vi "Analyze Frequency Response.vi"(0 "Per-Frequency Per-Site Waveform In":waveform(dbl)[][](array[waveform]), 5 "Frequency (Hz)":dbl[](array[numeric]), 7 "Window(Rectangle)":T1(ring), 11 "error in (no error)":errorcluster) -> (4 "DC values(V)":dbl[][](array[numeric]), 6 "detected amplitudes(Unit Peak)":dbl[][](array[numeric]), 8 "detected phases (deg)":dbl[][](array[numeric]), 10 "THD(%)":dbl[][](array[numeric]), 15 "error out":errorcluster)   [LabVIEW 2020]
doc: "This Vi helps to calculate the frequency response such as Amplitude, THD, Phase and DC Offset for the DUT or Ref_Mic"
uses:
  <vilib>/measure/matone.llb/Harmonic Distortion Analyzer N Chan.vi
  <vilib>/measure/matone.llb/Extract Single Tone Information N Chan.vi
  <vilib>/measure/madcrms.llb/Basic Averaged DC-RMS for N Chan.vi
  <vilib>/measure/NI_MAPro.lvlib
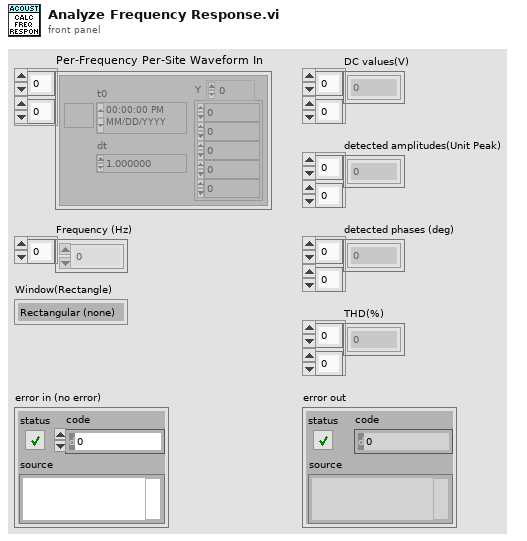
[diagram p1: front panel]
types:
  T1 = enum16{"Rectangular (none)", "Hanning", "Low side lobe"}
  T2 = cluster{"approx freq. (optional)":dbl, "search (+/- % of Fsampl.)":dbl}
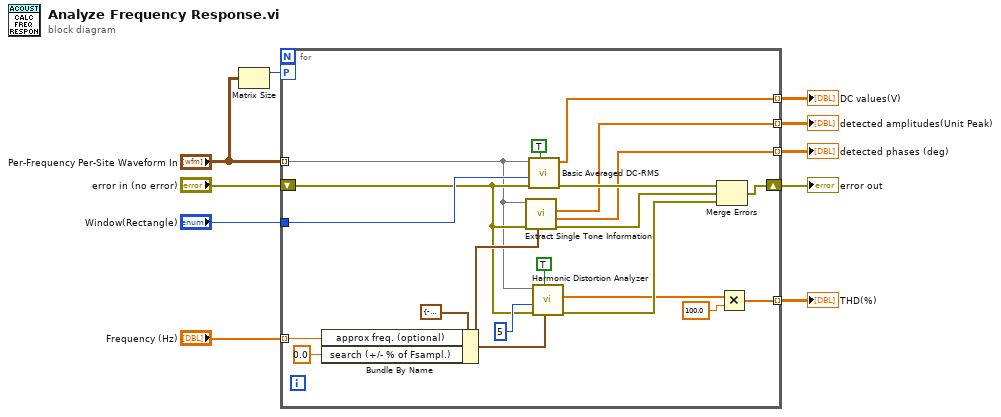
[diagram p0: block diagram]
diagram:
  n1 = Matrix Size(0:"Per-Frequency Per-Site Waveform In") -> (1:w1:i32)  [unwired: 1 out]
  n2 = for {
    tunnel: "Window(Rectangle)" -> [w25]
    shift-right: [w17] -> w8
    shift-left: "error in (no error)" -> [w23]
    tunnel: "Frequency (Hz)" -> [w21] mode=indexing
    tunnel: "Per-Frequency Per-Site Waveform In" -> [w22] mode=indexing
    tunnel: [w16] -> w6 mode=indexing
    tunnel: [w15] -> w5 mode=indexing
    tunnel: [w14] -> w4 mode=indexing
    tunnel: [w11] -> w3 mode=indexing
    workers-P: w1 -> [_]
    n3 = Bundle By Name(cluster=T2 {"approx freq. (optional)"=-1.0, "search (+/- % of Fsampl.)"=5.0} ("advanced search"), "approx freq. (optional)"=w21, "search (+/- % of Fsampl.)"=0.0) -> (w26:T2)
    n4 = call-poly <vilib>:"Extract Single Tone Information.vi"("advanced search"=w26, "error in (no error)"=w23, "time signals in"=w22) -> ("error out"=w19:errorcluster, "detected phases (deg)"=w14:dbl[], "detected amplitudes"=w15:dbl[])  [unwired: 3 in, 3 out]
    n5 = call-poly <vilib>:"Basic Averaged DC-RMS.vi"("reset"=TRUE, "error in (no error)"=w23, "window"=w25, "signals in"=w22) -> ("error out"=w20:errorcluster, "DC values"=w16:dbl[])  [unwired: 4 in, 2 out]
    n6 = call-poly <vilib>:"Harmonic Distortion Analyzer.vi"("advanced search"=w26, "stop search at Nyquist"=TRUE, "error in (no error)"=w23, "highest harmonic"=5, "signals in"=w22) -> ("error out"=w18:errorcluster, "THD"=w12:dbl[])  [unwired: 1 in, 4 out]
    n7 = Merge Errors(w20, w19, w18) -> (w17:errorcluster)
    n8 = Multiply(x=w12, y=100.0) -> (x*y=w11:dbl[])
  }
  "error out" <- w8
  "DC values(V)" <- w6
  "detected amplitudes(Unit Peak)" <- w5
  "detected phases (deg)" <- w4
  "THD(%)" <- w3
